vi "Parse Set Delimiter.vi"(8 "Error In":errorcluster) -> (0 "Error Out":errorcluster)   [LabVIEW 2018, in "Tests.lvlib" / "Lexer.lvlib"]
uses:
  Lexer.lvlib
  src/Toolkit/Low-Level/Support/Lex String.vi
  <vilib>/addons/_JKI Toolkits/Caraya/classes/Test/Test.lvclass
  <vilib>/addons/_JKI Toolkits/Caraya/classes/Assert/Assert.lvclass
  src/Toolkit/Toolkit.lvlib
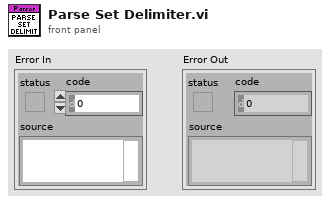
[diagram p1: front panel]
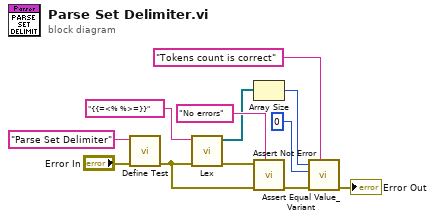
[diagram p0: block diagram]
diagram:
  n1 = call <vilib>:"Define Test.vi"("error in (no error)"="Error In", "Label (VI Title)"="Parse Set Delimiter") -> ("error out"=w1:errorcluster)  [unwired: 9 in]
  n2 = call-poly "Lex.vi"("Error In"=w1, "Input"="{{=<% %>=}}" ("format string")) -> ("Error Out"=w10:errorcluster, "Tokens"=w4:refnum<class "Abstract.lvclass">[])  [unwired: 8 in]
  n3 = Array Size(array=w4) -> (size(s)=w6:i32)
  n4 = call <vilib>:"Assert Not Error.vi"("Label"="No errors", "error in (no error)"=w1, "Not Error?"=w10) -> ("error out"=w8:errorcluster)  [unwired: 8 in]
  n5 = call <vilib>:"Assert Equal Value_Variant.vi"("Label"="Tokens count is correct", "error in (no error)"=w8, "Y"=0 ("size(s)"), "X"=w6) -> ("error out"=→"Error Out":errorcluster)  [unwired: 7 in]
